vi "Main.vi"() -> ()   [LabVIEW 2017]
doc: "The myRIO Project template acquires acceleration data from the onboard accelerometer and displays the changes of acceleration values in a waveform chart."
uses:
  <vilib>/myRIO/Instrument Drivers/Onboard IO/I2C/typedefs/I2C User Configuration.ctl
  <vilib>/myRIO/Instrument Drivers/Onboard IO/I2C/typedefs/I2C Transfer Rate.ctl
  <vilib>/Platform/TimedLoop/XDataNode/timing_clust.ctl
  <vilib>/Platform/TimedLoop/XDataNode/nitl_modes.ctl
  <vilib>/Platform/TimedLoop/XDataNode/wakeup.ctl
  <vilib>/myRIO/Instrument Drivers/Onboard IO/DIO/typedefs/DIO Reference.ctl
  <vilib>/myRIO/Common/Instrument Driver Framework/Utilities/typedefs/myRIO Generic Hardware Reference.ctl
  <vilib>/myRIO/Common/Instrument Driver Framework/Utilities/typedefs/Hardware Version Enum.ctl
  <vilib>/myRIO/Common/Instrument Driver Framework/Utilities/typedefs/myRIO v1.0 Reference.ctl
  <vilib>/myRIO/Common/Instrument Driver Framework/Utilities/typedefs/Generic FPGA Reference.ctl
  <vilib>/myRIO/Common/Instrument Driver Framework/myRIO v1.0/DIO/typedefs/DIO Channels List.ctl
  <vilib>/myRIO/Common/Instrument Driver Framework/myRIO v1.0/DIO/typedefs/DIO Channels Enum.ctl
  <vilib>/userdefined/High Color/nirio_resource_hc.ctl
  <vilib>/myRIO/Common/Instrument Driver Framework/myRIO v1.0/Encoder/typedefs/Encoder Signal Mode.ctl
  <vilib>/myRIO/Instrument Drivers/Onboard IO/Encoder/typedefs/Encoder Reference.ctl
  <vilib>/myRIO/Common/Instrument Driver Framework/myRIO v1.0/Encoder/typedefs/Encoder Channels Enum.ctl
  <vilib>/myRIO/Common/Instrument Driver Framework/myRIO v1.0/Encoder/typedefs/Encoder Configuration v1.0.ctl
  <vilib>/myRIO/Instrument Drivers/Onboard IO/PWM/typedefs/PWM Reference.ctl
  <vilib>/myRIO/Common/Instrument Driver Framework/myRIO v1.0/PWM/typedefs/PWM Channels Enum.ctl
  <vilib>/myRIO/Instrument Drivers/Onboard IO/PWM/typedefs/PWM Configuration.ctl
  <vilib>/myRIO/Common/Instrument Driver Framework/Utilities/vis/Is FPGA Ref Available.vi
  <vilib>/myRIO/Common/Instrument Driver Framework/myRIO v1.0/Encoder/vis/myRIO v1.1 Open Encoder.vi
  <vilib>/myRIO/Common/Instrument Driver Framework/myRIO v1.0/DIO/vis/myRIO v1.1 Open DIO.vi
  <vilib>/myRIO/Common/Instrument Driver Framework/myRIO v1.0/PWM/vis/myRIO v1.1 Open PWM.vi
  <vilib>/myRIO/Instrument Drivers/Onboard IO/PWM/vis/Set Duty Cycle and Frequency.vi
  <vilib>/myRIO/Common/Instrument Driver Framework/Utilities/vis/Validate Channels.vi
  <vilib>/myRIO/Common/Instrument Driver Framework/myRIO v1.0/Encoder/vis/myRIO v1.0 Reserve Encoder.vi
  <vilib>/myRIO/Common/Instrument Driver Framework/myRIO v1.0/DIO/vis/myRIO v1.0 Reserve DIO.vi
  <vilib>/myRIO/Common/Instrument Driver Framework/myRIO v1.0/PWM/vis/myRIO v1.0 Reserve PWM.vi
  <vilib>/myRIO/Common/Instrument Driver Framework/myRIO v1.0/UART/vis/myRIO v1.0 Close UART.vi
  <vilib>/myRIO/Common/Instrument Driver Framework/myRIO v1.0/I2C/vis/myRIO v1.1 Open I2C.vi
  <vilib>/myRIO/Common/Instrument Driver Framework/myRIO v1.0/Encoder/vis/myRIO v1.0 Build MUX Configuration Encoder.vi
  <vilib>/myRIO/Common/Instrument Driver Framework/myRIO v1.0/Resource Manager/vis/myRIO v1.0 Reserve Channel List.vi
  <vilib>/myRIO/Common/Instrument Driver Framework/myRIO v1.0/DIO/vis/myRIO v1.0 Build MUX Configuration DIO.vi
  <vilib>/myRIO/Common/Instrument Driver Framework/myRIO v1.0/PWM/vis/myRIO v1.0 Build MUX Configuration PWM.vi
  <vilib>/myRIO/Common/Instrument Driver Framework/myRIO v1.0/I2C/vis/myRIO v1.0 Reserve I2C.vi
  <vilib>/myRIO/Common/Instrument Driver Framework/myRIO v1.0/Resource Manager/vis/myRIO v1.0 Create Configuration List.vi
  <vilib>/myRIO/Common/Instrument Driver Framework/myRIO v1.0/Resource Manager/vis/myRIO v1.0 Reserve Channel.vi
  <vilib>/myRIO/Common/Instrument Driver Framework/myRIO v1.0/Resource Manager/vis/myRIO v1.0 Unreserve Channel.vi
  <vilib>/myRIO/Common/Instrument Driver Framework/myRIO v1.0/I2C/vis/myRIO v1.0 Build MUX Configuration I2C.vi
  <vilib>/myRIO/Common/Instrument Driver Framework/myRIO v1.0/Resource Manager/vis/myRIO v1.0 Build Mutex Name.vi
  <vilib>/Utility/VariantDataType/GetNumericInfo.vi
  <vilib>/Utility/error.llb/Error Cluster From Error Code.vi
  <vilib>/myRIO/Common/Instrument Driver Framework/myRIO v1.0/myRIO v1.1 Open.vi
  <vilib>/myRIO/Common/Instrument Driver Framework/Utilities/vis/IO Manager.vi
  <vilib>/myRIO/Common/Instrument Driver Framework/Utilities/vis/Configuration Manager.vi
  <vilib>/myRIO/Common/Instrument Driver Framework/myRIO v1.0/Resource Manager/vis/myRIO v1.0 Configure IO.vi
  <vilib>/myRIO/Common/Instrument Driver Framework/myRIO v1.0/myRIO v1.0 Close.vi
  <vilib>/myRIO/Common/Instrument Driver Framework/myRIO v1.0/I2C/vis/myRIO v1.0 Configure I2C.vi
  <vilib>/myRIO/Common/Instrument Driver Framework/myRIO v1.0/I2C/vis/myRIO v1.0 Write I2C.vi
  <vilib>/myRIO/Common/Instrument Driver Framework/myRIO v1.0/DIO/vis/myRIO v1.0 Read DIO.vi
  <vilib>/myRIO/Common/Instrument Driver Framework/myRIO v1.0/DIO/vis/myRIO v1.0 Write DIO.vi
  <vilib>/myRIO/Common/Instrument Driver Framework/myRIO v1.0/I2C/vis/myRIO v1.0 Read I2C.vi
  <vilib>/myRIO/Common/Instrument Driver Framework/Utilities/vis/FPGA Ref Manager.vi
  <vilib>/myRIO/Common/Instrument Driver Framework/myRIO v1.0/myRIO v1.0 Reset FPGA.vi
  <vilib>/myRIO/Common/Instrument Driver Framework/myRIO v1.0/IRQ/vis/myRIO v1.0 IRQ Info FGV.vi
  <vilib>/myRIO/Common/Instrument Driver Framework/myRIO v1.0/IRQ/vis/myRIO v1.0 Timer IRQ Info FGV.vi
  <vilib>/myRIO/Common/Instrument Driver Framework/myRIO v1.0/IRQ/vis/myRIO v1.0 ISR Agent.vi
  <vilib>/myRIO/Common/Instrument Driver Framework/myRIO v1.0/Encoder/vis/myRIO v1.0 Configure Encoder.vi
  <vilib>/myRIO/Common/Instrument Driver Framework/myRIO v1.0/Encoder/vis/myRIO v1.0 Read Encoder.vi
  <vilib>/myRIO/Common/Instrument Driver Framework/myRIO v1.0/PWM/vis/myRIO v1.0 Write PWM.vi
  <vilib>/platform/TimedLoop/XDataNode/XDataNode.xnode
  <vilib>/myRIO/Express VI/Onboard IO/DO/DO Express VI.xnode
  <vilib>/myRIO/Instrument Drivers/Onboard IO/DIO/vis/myRIO DIO Open.xnode
  <vilib>/myRIO/Express VI/Onboard IO/Encoder/Encoder Express VI.xnode
  <vilib>/myRIO/Common/Instrument Driver Framework/myRIO v1.0/Encoder/typedefs/Encoder Count Direction Enum.ctl
  <vilib>/myRIO/Instrument Drivers/Onboard IO/Encoder/vis/myRIO Encoder Open.xnode
  <vilib>/myRIO/Express VI/Onboard IO/PWM/PWM Express VI.xnode
  <vilib>/myRIO/Instrument Drivers/Onboard IO/PWM/vis/myRIO PWM Open.xnode
  <vilib>/myRIO/Instrument Drivers/Utilities/Utilities.lvlib
  <vilib>/myRIO/Instrument Drivers/Onboard IO/I2C/I2C.lvlib
  <vilib>/myRIO/Instrument Drivers/Onboard IO/DIO/DIO.lvlib
  <vilib>/Platform/TimedLoop/XDataNode/XDNodeRunTimeDep.lvlib
  <vilib>/ptbypt/NI_PtbyPt.lvlib
  <vilib>/myRIO/Instrument Drivers/Onboard IO/Encoder/Encoder.lvlib
  <vilib>/myRIO/Instrument Drivers/Onboard IO/PWM/PWM.lvlib
panel:
  out "Led":bool
  in  "[ESC]":bool
  out "X":i16
  out "Y":i16
  out "Z":i16
  out "DATA":u8[](array[numeric]) format="%02x"
  out "Waveform Chart":cluster{i16, i16, i16}(graph)
  out "INT_SOURCE":bool[](array[boolean])
  out "error out":errorcluster
  in  "Stop":bool
  in  "(PWM Duty %)":dbl(slide)=1.0 scale=1.0..0.3
  in  "Direction":bool caption="Dirección"
  in  "Reseteo del contador":bool
  out "Contador":i32 format="%1d"
  out "Dirección":enum16{"Counting Up", "Counting Down"}(ring)
  in  "[ESC] 2":bool
  out "X rate":i16
  out "Y rate":i16
  out "Z rate":i16
  out "DATA 2":u8[](array[numeric]) format="%02x"
  out "Angular rate [LSB/sec]":cluster{i16, i16, i16}(graph)
  out "Angular displacement [LSB]":T1(graph)
  out "X displacement":dbl format="%#_5g"
  out "Y displacement":dbl format="%#_5g"
  out "Z displacement":dbl format="%#_5g"
  in  "reset integrator":bool
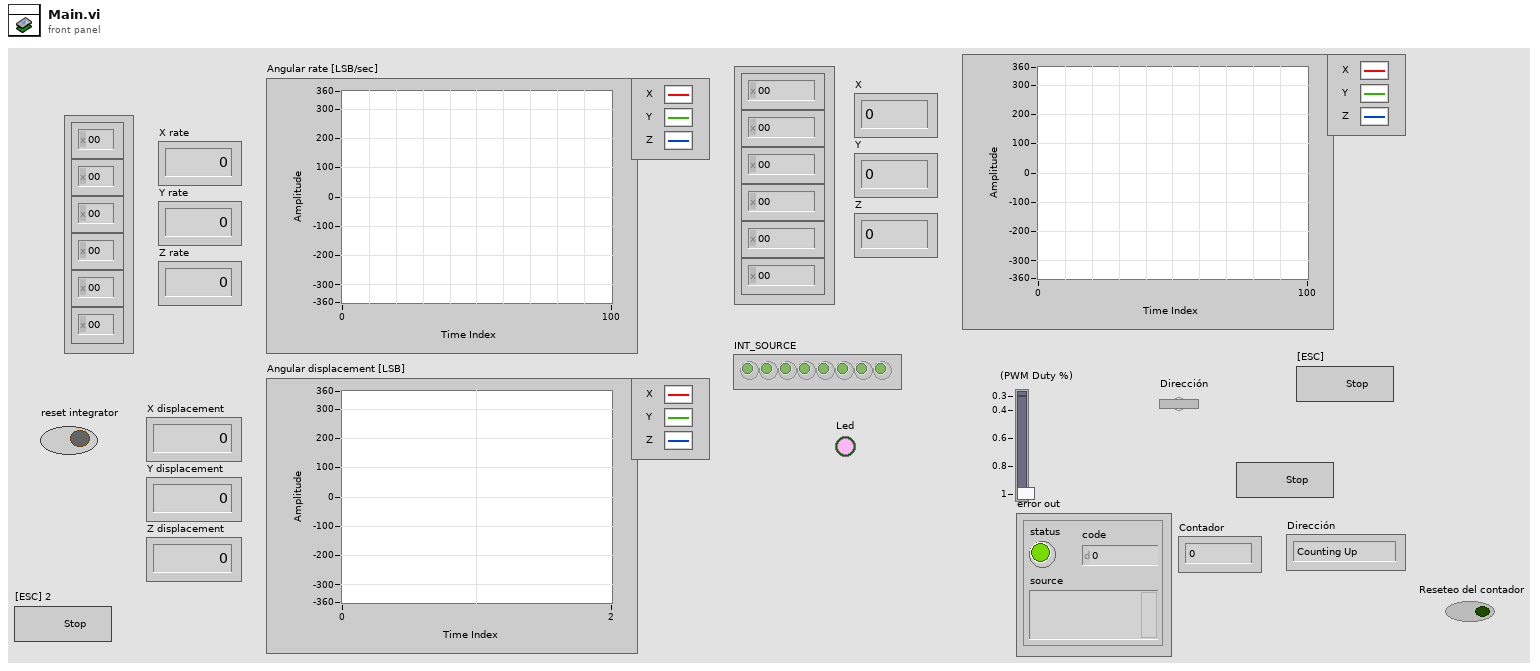
[diagram p1: front panel]
types:
  T1 = cluster{"integral x(t)":dbl, "integral x(t)":dbl, "integral x(t)":dbl}
  T2 = typedef "I2C.lvlib/I2C User Configuration.ctl" = cluster{"I2C Transfer Rate":T3}
  T3 = typedef "I2C.lvlib/I2C Transfer Rate.ctl" = enum16{"Standard mode (100 kbps)", "Fast mode (400 kbps)"}
  T4 = typedef "Encoder.lvlib/Encoder Reference.ctl" = cluster{"myRIO Reference":T5, "Encoder Channels Enum":T9}
  T5 = typedef "myRIO Generic Hardware Reference.ctl" = cluster{"myRIO Model":T6, "myRIO Hardware Reference":T7}
  T6 = typedef "Hardware Version Enum.ctl" = enum16{"Unknown", "myRIO-1900", "myRIO-1950", "roboRIO", "NI ELVIS RIO CM"}
  T7 = typedef "myRIO v1.0 Reference.ctl" = cluster{"Generic FPGA Reference":T8, "Allow multiple opens":bool}
  T8 = typedef "Generic FPGA Reference.ctl" = refnum<k20>
  T9 = typedef "Encoder Channels Enum.ctl" = enum16{"Not Connected", "C/ENC0", "C/ENC1", "A/ENC", "B/ENC", "DIO/ENC0", "DIO/ENC1", "DIO/ENC2", "DIO/ENC3", "DIO/ENC4"}
  T10 = typedef "Encoder Signal Mode.ctl" = enum16{"Quadrature phase signal", "Step and direction signal"}
  T11 = typedef "nirio_resource_hc.ctl" = tag
  T12 = typedef "DIO.lvlib/DIO Reference.ctl" = cluster{"myRIO Reference":T5, "DIO Channels List":T13}
  T13 = typedef "DIO Channels List.ctl" = T14[]
  T14 = typedef "DIO Channels Enum.ctl" = enum16{"Not Connected", "C/DIO0", "C/DIO1", "C/DIO2", "C/DIO3", "C/DIO4", "C/DIO5", "C/DIO6", "C/DIO7", "A/DIO0", "A/DIO1", "A/DIO2", "A/DIO3", "A/DIO4", "A/DIO5", "A/DIO6", "A/DIO7", "A/DIO8", "A/DIO9", "A/DIO10", "A/DIO11", "A/DIO12", "A/DIO13", "A/DIO14", "A/DIO15", "B/DIO0", "B/DIO1", "B/DIO2", "B/DIO3", "B/DIO4", "B/DIO5", "B/DIO6", "B/DIO7", "B/DIO8", "B/DIO9", "B/DIO10", "B/DIO11", "B/DIO12", "B/DIO13", "B/DIO14", "B/DIO15", "LED0", "LED1", "LED2", "LED3", "Button0", "DIO/DIO0", "DIO/DIO1", "DIO/DIO2", "DIO/DIO3", "DIO/DIO4", "DIO/DIO5", "DIO/DIO6", "DIO/DIO7", "DIO/DIO8", "DIO/DIO9", "SPI/CS0", "SPI/CS1", "SPI/CS2", "SPI/CS3", "LED RADIO (Green)", "LED RADIO (Red)", "LED COMM (Green)", "LED COMM (Red)", "LED MODE (Green)", "LED MODE (Red)"}
  T15 = typedef "PWM.lvlib/PWM Reference.ctl" = cluster{"myRIO Reference":T5, "PWM Channels Enum":T16, "PWM Configuration":T17}
  T16 = typedef "PWM Channels Enum.ctl" = enum16{"Not Connected", "C/PWM0", "C/PWM1", "A/PWM0", "A/PWM1", "A/PWM2", "B/PWM0", "B/PWM1", "B/PWM2", "PWM/PWM0", "PWM/PWM1", "PWM/PWM2", "PWM/PWM3", "PWM/PWM4", "PWM/PWM5", "PWM/PWM6", "PWM/PWM7", "PWM/PWM8", "PWM/PWM9"}
  T17 = typedef "PWM.lvlib/PWM Configuration.ctl" = cluster{"Frequency":dbl, "Duty Cycle":dbl}
  T18 = typedef "Encoder Count Direction Enum.ctl" = enum16{"Counting Up", "Counting Down"}
  T19 = typedef "I2C.lvlib/I2C Reference.ctl" = cluster{"myRIO Reference":T5, "I2C Channels Enum":T20, "I2C Configuration":T21}
  T20 = typedef "I2C Channels Enum.ctl" = enum16{"Not Connected", "A/I2C", "B/I2C", "I2C/I2C"}
  T21 = typedef "I2C.lvlib/I2C Configuration.ctl" = cluster{"I2C Transfer Rate":T3}
  T22 = typedef "XDNodeRunTimeDep.lvlib/timing_clust.ctl" = cluster{"Expected End [f-1]":u64, "Actual End [f-1]":u64, "Finished Late? [f-1]":bool, "Expected End [i-1]":u64, "Actual End [i-1]":u64, "Finished Late? [i-1]":bool, "Expected Start [i]":u64, "Actual Start [i]":u64, "Expected Start [f]":u64, "Actual Start [f]":u64, "Source Name":string, "Structure Name":string, "Period":i64, "Deadline":i64, "Offset":i64, "Start":i64, "Priority":i32, "Timeout":i32, "Mode":T23, "Wakeup Reason":T24, "Error":errorcluster, "Source Type":string, "Secondary Source Type":string, "Global End Time":u64, "Global Start Time":u64, "Frame Duration":u64, "Iteration Duration":u64, "Assigned CPU":i32, "I/O Scan Engine Mode":u32}
  T23 = typedef "XDNodeRunTimeDep.lvlib/nitl_modes.ctl" = enum32{"No Change", "Process missed periods, maintain original phase", "Discard missed periods, maintain original phase", "Process missed periods, ignore original phase", "Discard missed periods, ignore original phase"}
  T24 = typedef "XDNodeRunTimeDep.lvlib/wakeup.ctl" = enum32{"Normal", "Aborted", "Asynchronous wakeup", "Timing source error", "Timed loop error", "Timeout"}
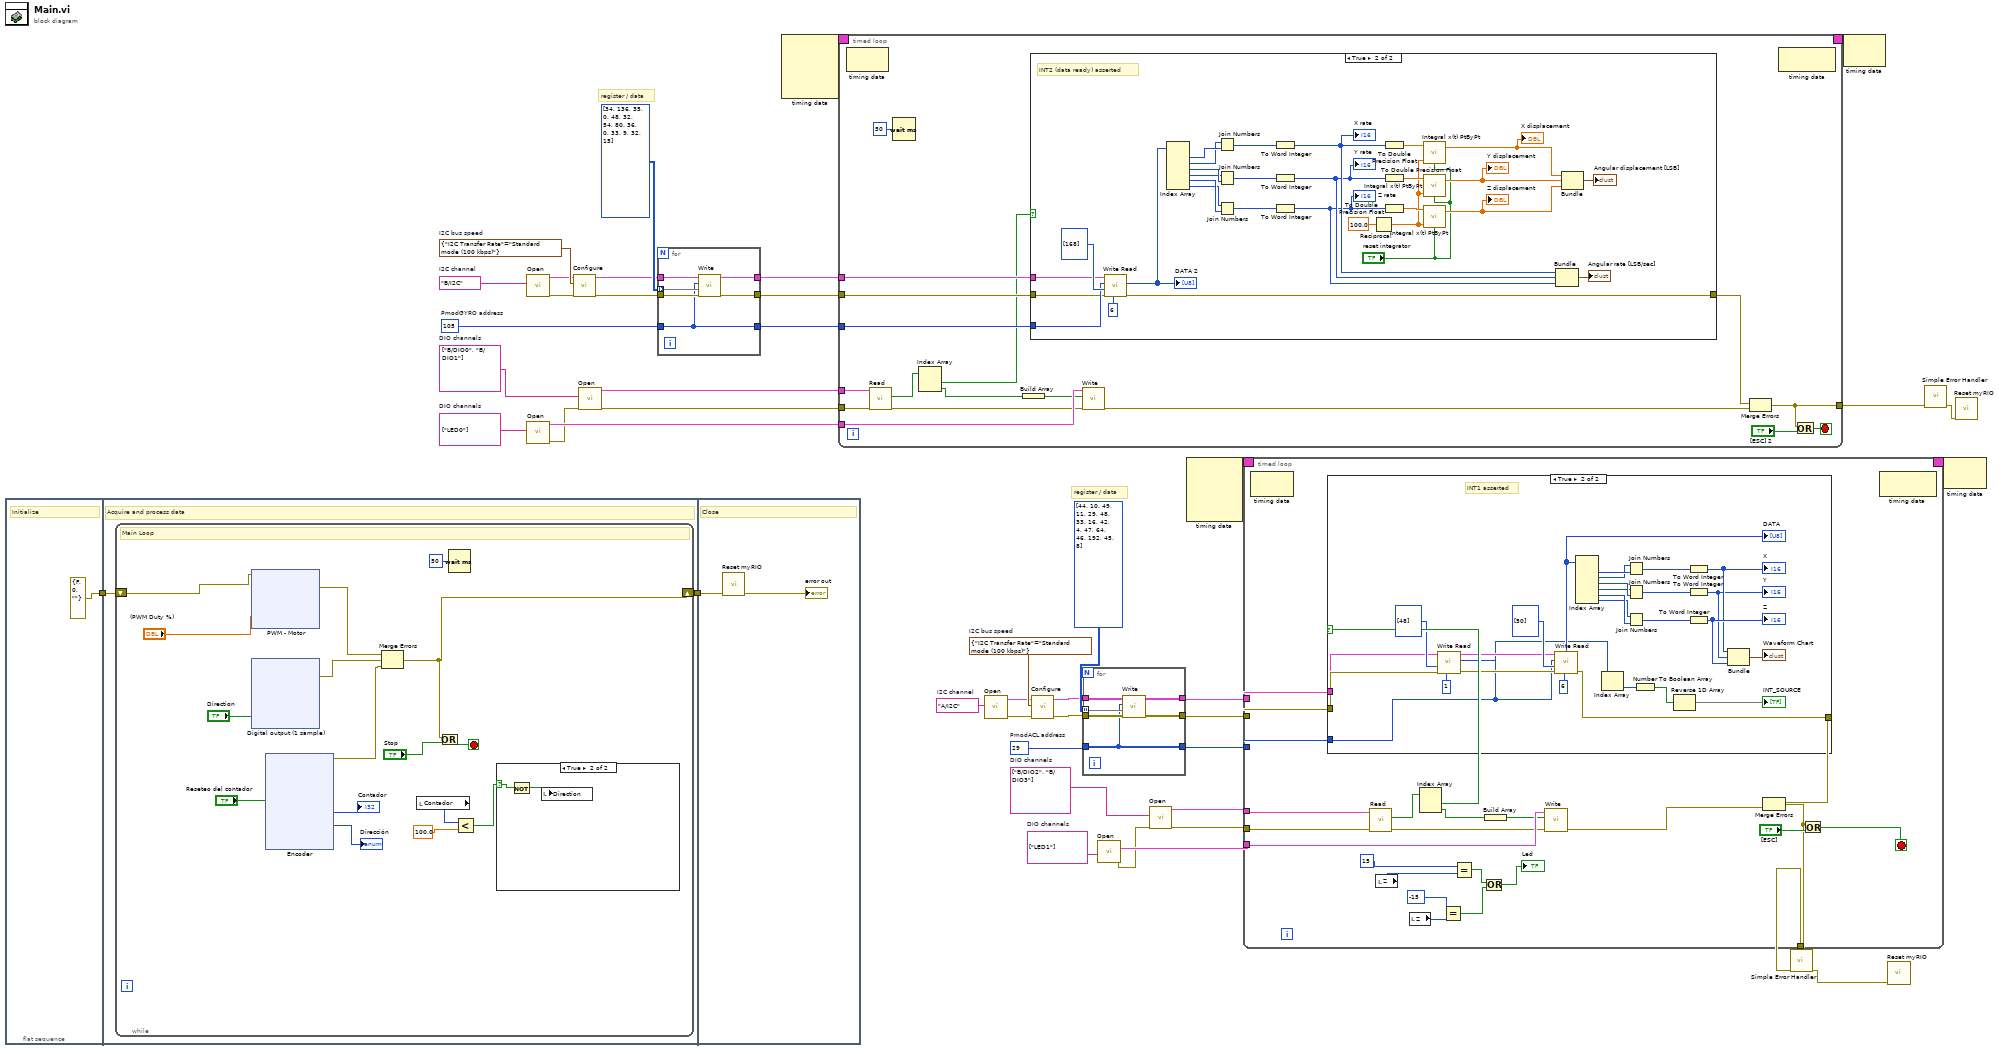
[diagram p0: block diagram]
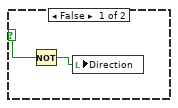
[diagram p3: hidden frame]
diagram:
  w3 = tag[] ["LED1"]  # DIO channels
  w4 = tag[] ["B/DIO2", "B/DIO3"]  # DIO channels
  w16 = T2 {"I2C Transfer Rate"=enum."Standard mode (100 kbps)"}  # I2C bus speed
  w17 = tag "A/I2C"  # I2C channel
  w7 = u8 29  # PmodACL address
  w26 = tag[] ["LED0"]  # DIO channels
  w27 = tag[] ["B/DIO0", "B/DIO1"]  # DIO channels
  w39 = T2 {"I2C Transfer Rate"=enum."Standard mode (100 kbps)"}  # I2C bus speed
  w40 = tag "B/I2C"  # I2C channel
  w30 = u8 105  # PmodGYRO address
  # "register / data"
  # "register / data"
  n1 = flat-sequence {
    tunnel: [errorcluster {"status"=FALSE, "code"=0, "source"=""} ("error in (no error)")] -> w23
    tunnel: w23 -> [w47]
    tunnel: [w46] -> w22
    tunnel: w22 -> [w185]
    frame #0 {
      # "Initialize"
    }
    frame #1 {
      # "Acquire and process data"
      n2 = while {
        shift-right: [w57] -> w46
        shift-left: w47 -> [w60]
        stop <- w62 stop-if-true
        # "Main Loop"
        n3 = xnode "PWM - Motor"("Duty Cycle"="(PWM Duty %)", "error in (no error)"=w60) -> ("error out"=w59:errorcluster)
        n4 = xnode "Digital output (1 sample)"("DIR0 (A/DIO6 (Pin 23))"="Direction") -> ("error out"=w58:errorcluster)  [unwired: 1 in]
        n5 = xnode "Encoder"("Reset Counter"="Reseteo del contador") -> ("Counter Value"=→"Contador":i32, "Counter Direction"=→"Dirección":T18, "error out"=w55:errorcluster)  [unwired: 1 in, 1 out]
        n6 = Merge Errors(w59, w58, w55) -> (w57:errorcluster)
        n7 = local read "Contador"() -> (w50:i32)
        n8 = Or(x=w57, y="Stop") -> (x .or. y?=w62:bool)
        n9 = Wait (ms)(milliseconds to wait=u32 50) -> ()  [unwired: 1 out]
        n10 = Less?(x=w50, y=100.0) -> (x < y?=w49:bool)
        n11 = case shown="True" w49 {
          selector: w49 -> [w64 w67]
          frame False {
            n12 = Not(x=w64) -> (.not. x?=w65:bool)
            n13 = local write "Direction"(w65) -> ()
          }
          frame True {
            n14 = Not(x=w67) -> (.not. x?=w66:bool)
            n15 = local write "Direction"(w66) -> ()
          }
        }
      }
    }
    frame #2 {
      # "Close"
      n16 = call <vilib>:"Reset myRIO.vi"("error in (no error)"=w185) -> ("error out"=→"error out":errorcluster)  [unwired: 10 in]
    }
  }
  n17 = call <vilib>:"Open.vi"("Channel Name"=w40) -> ("error out"=w37:errorcluster, "I2C Ref Out"=w38:T19)  [unwired: 9 in]
  n18 = call <vilib>:"Open.vi"("Channel Names"=w26) -> ("error out"=w24:errorcluster, "DIO Ref Out"=w25:T12)  [unwired: 9 in]
  n19 = call <vilib>:"Configure.vi"("error in (no error)"=w37, "I2C User Configuration"=w39, "I2C Ref In"=w38) -> ("error out"=w31:errorcluster, "I2C Ref Out"=w32:T19)  [unwired: 7 in]
  n20 = call <vilib>:"Open.vi"("error in (no error)"=w24, "Channel Names"=w27) -> ("error out"=w29:errorcluster, "DIO Ref Out"=w28:T12)  [unwired: 8 in]
  n21 = for {
    tunnel: [w191] -> w36
    tunnel: [w190] -> w35
    tunnel: [w186] -> w34
    tunnel: u8[][] [[34, 136], [35, 0], [48, 32], [54, 80], [36, 0], [33, 9], [32, 15]] ("Bytes to Write") -> [w189] mode=indexing
    tunnel: w32 -> [w188]
    tunnel: w31 -> [w187]
    tunnel: w30 -> [w186]
    n22 = call <vilib>:"Write.vi"("error in (no error)"=w187, "Bytes to Write"=w189, "Slave Address (7-bit)"=w186, "I2C Ref In"=w188) -> ("error out"=w191:errorcluster, "I2C Ref Out"=w190:T19)  [unwired: 6 in]
  }
  n23 = node-c288() -> (w44:T22)  [unwired: 4 in]
  n24 = timed-loop {
    tunnel: [w193] -> w41
    tunnel: w34 -> [w204]
    tunnel: w36 -> [w206]
    tunnel: w35 -> [w205]
    tunnel: w29 -> [w203]
    tunnel: w28 -> [w202]
    timing: w44 -> [_]
    timing-out: [_] -> w43
    tunnel: w25 -> [w198]
    stop <- w208 stop-if-true
    n25 = node-c288() -> ()  [unwired: 1 in, 1 out]
    n26 = call <vilib>:"Read.vi"("error in (no error)"=w203, "DIO Ref In"=w202) -> ("error out"=w197:errorcluster, "Values"=w199:bool[])  [unwired: 7 in, 1 out]
    n27 = Wait (ms)(milliseconds to wait=u32 50) -> ()  [unwired: 1 out]
    n28 = Index Array "Index Array"(array=w199) -> (element #1=w200:bool, element #2=w195:bool)  [unwired: 2 in]
    n29 = Build Array "Build Array"(w195) -> (w196:bool[])
    n30 = case shown="True" w200 {
      tunnel: w206 -> [w211 w219]
      tunnel: w205 -> [_ w220]
      tunnel: w204 -> [_ w229]
      tunnel: [w211 w228] -> w201
      frame False {
        # "INT2 (data ready) deasserted"
      }
      frame True {
        # "INT2 (data ready) asserted"
        n31 = call <vilib>:"Write Read.vi"("Byte Count"=u32 6, "error in (no error)"=w219, "Bytes to Write"=u8[] [168], "Slave Address (7-bit)"=w229, "I2C Ref In"=w220) -> ("error out"=w228:errorcluster, "Bytes Read"=w227:u8[])  [unwired: 3 in, 1 out]
        "DATA 2" <- w227
        n32 = Index Array "Index Array"(array=w227) -> (element #1=w237:u8, element #2=w236:u8, element #3=w235:u8, element #4=w234:u8, element #5=w233:u8, element #6=w232:u8)  [unwired: 6 in]
        n33 = Join Numbers(hi=w236, lo=w237) -> ((hi.lo)=w241:u16)
        n34 = Join Numbers(hi=w234, lo=w235) -> ((hi.lo)=w240:u16)
        n35 = Join Numbers(hi=w232, lo=w233) -> ((hi.lo)=w239:u16)
        n36 = To Word Integer(number=w241) -> (16bit integer=w226:i16)
        "X rate" <- w226
        n37 = To Word Integer(number=w240) -> (16bit integer=w222:i16)
        "Y rate" <- w222
        n38 = To Word Integer(number=w239) -> (16bit integer=w221:i16)
        "Z rate" <- w221
        n39 = Reciprocal(x=100.0 ("dt")) -> (1/x=w217:dbl)
        n40 = To Double Precision Float(number=w226) -> (double precision float=w212:dbl)
        n41 = To Double Precision Float(number=w222) -> (double precision float=w225:dbl)
        n42 = To Double Precision Float(number=w221) -> (double precision float=w224:dbl)
        n43 = call <vilib>:"Integral x(t) PtByPt.vi"("initialize"="reset integrator", "dt"=w217, "x"=w212) -> ("integral x(t)"=w213:dbl)  [unwired: 1 in, 1 out]
        "X displacement" <- w213
        n44 = call <vilib>:"Integral x(t) PtByPt.vi"("initialize"="reset integrator", "dt"=w217, "x"=w225) -> ("integral x(t)"=w216:dbl)  [unwired: 1 in, 1 out]
        "Y displacement" <- w216
        n45 = call <vilib>:"Integral x(t) PtByPt.vi"("initialize"="reset integrator", "dt"=w217, "x"=w224) -> ("integral x(t)"=w215:dbl)  [unwired: 1 in, 1 out]
        "Z displacement" <- w215
        n46 = Bundle "Bundle"(w226, w222, w221) -> (→"Angular rate [LSB/sec]":cluster{i16, i16, i16})  [unwired: 1 in]
        n47 = Bundle "Bundle"("integral x(t)"=w213, "integral x(t)"=w216, "integral x(t)"=w215) -> (→"Angular displacement [LSB]":T1)  [unwired: 1 in]
      }
    }
    n48 = call <vilib>:"Write.vi"("error in (no error)"=w197, "Values"=w196, "DIO Ref In"=w198) -> ("error out"=w194:errorcluster)  [unwired: 6 in, 1 out]
    n49 = Merge Errors "Merge Errors"(w201, w194) -> (w193:errorcluster)
    n50 = node-c288() -> ()  [unwired: 1 in, 1 out]
    n51 = Or(x=w193, y="[ESC] 2") -> (x .or. y?=w208:bool)
  }
  n52 = call <vilib>:"Open.vi"("Channel Name"=w17) -> ("error out"=w14:errorcluster, "I2C Ref Out"=w15:T19)  [unwired: 9 in]
  n53 = call <vilib>:"Configure.vi"("error in (no error)"=w14, "I2C User Configuration"=w16, "I2C Ref In"=w15) -> ("error out"=w8:errorcluster, "I2C Ref Out"=w9:T19)  [unwired: 7 in]
  n54 = for {
    tunnel: [w247] -> w13
    tunnel: [w246] -> w12
    tunnel: [w242] -> w11
    tunnel: u8[][] [[44, 10], [49, 11], [29, 48], [33, 16], [42, 4], [47, 64], [46, 192], [45, 8]] ("Bytes to Write") -> [w245] mode=indexing
    tunnel: w9 -> [w244]
    tunnel: w8 -> [w243]
    tunnel: w7 -> [w242]
    n55 = call <vilib>:"Write.vi"("error in (no error)"=w243, "Bytes to Write"=w245, "Slave Address (7-bit)"=w242, "I2C Ref In"=w244) -> ("error out"=w247:errorcluster, "I2C Ref Out"=w246:T19)  [unwired: 6 in]
  }
  n56 = call <vilib>:"Open.vi"("Channel Names"=w3) -> ("error out"=w1:errorcluster, "DIO Ref Out"=w2:T12)  [unwired: 9 in]
  n57 = call <vilib>:"Open.vi"("error in (no error)"=w1, "Channel Names"=w4) -> ("error out"=w6:errorcluster, "DIO Ref Out"=w5:T12)  [unwired: 8 in]
  n58 = node-c288() -> (w21:T22)  [unwired: 4 in]
  n59 = timed-loop {
    tunnel: [w255] -> w18
    tunnel: w11 -> [w266]
    tunnel: w13 -> [w268]
    tunnel: w12 -> [w267]
    tunnel: w6 -> [w265]
    tunnel: w5 -> [w264]
    timing: w21 -> [_]
    timing-out: [_] -> w20
    tunnel: w2 -> [w260]
    stop <- w270 stop-if-true
    n60 = node-c288() -> ()  [unwired: 1 in, 1 out]
    n61 = call <vilib>:"Read.vi"("error in (no error)"=w265, "DIO Ref In"=w264) -> ("error out"=w259:errorcluster, "Values"=w261:bool[])  [unwired: 7 in, 1 out]
    n62 = local read "Z"() -> (w254:i16)
    n63 = local read "Z"() -> (w252:i16)
    n64 = Index Array "Index Array"(array=w261) -> (element #1=w262:bool, element #2=w257:bool)  [unwired: 2 in]
    n65 = case shown="True" w262 {
      tunnel: w268 -> [w273 w292]
      tunnel: w267 -> [_ w291]
      tunnel: w266 -> [_ w280]
      tunnel: [w273 w276] -> w263
      frame False {
        # "INT1 deasserted"
      }
      frame True {
        # "INT1 asserted"
        n66 = call <vilib>:"Write Read.vi"("Byte Count"=u32 1, "error in (no error)"=w292, "Bytes to Write"=u8[] [48], "Slave Address (7-bit)"=w280, "I2C Ref In"=w291) -> ("error out"=w281:errorcluster, "Bytes Read"=w274:u8[], "I2C Ref Out"=w282:T19)  [unwired: 3 in]
        n67 = call <vilib>:"Write Read.vi"("Byte Count"=u32 6, "error in (no error)"=w281, "Bytes to Write"=u8[] [50], "Slave Address (7-bit)"=w280, "I2C Ref In"=w282) -> ("error out"=w276:errorcluster, "Bytes Read"=w275:u8[])  [unwired: 3 in, 1 out]
        "DATA" <- w275
        n68 = Index Array "Index Array"(array=w275) -> (element #1=w290:u8, element #2=w289:u8, element #3=w288:u8, element #4=w287:u8, element #5=w286:u8, element #6=w285:u8)  [unwired: 6 in]
        n69 = Index Array "Index Array"(array=w274) -> (element=w279:u8)  [unwired: 1 in]
        n70 = Join Numbers(hi=w289, lo=w290) -> ((hi.lo)=w301:u16)
        n71 = Join Numbers(hi=w287, lo=w288) -> ((hi.lo)=w300:u16)
        n72 = Join Numbers(hi=w285, lo=w286) -> ((hi.lo)=w299:u16)
        n73 = Number To Boolean Array(number=w279) -> (Boolean array=w278:bool[])
        n74 = Reverse 1D Array(array=w278) -> (reversed array=→"INT_SOURCE":bool[])
        n75 = To Word Integer(number=w301) -> (16bit integer=w296:i16)
        "X" <- w296
        n76 = To Word Integer(number=w300) -> (16bit integer=w295:i16)
        "Y" <- w295
        n77 = To Word Integer(number=w299) -> (16bit integer=w298:i16)
        "Z" <- w298
        n78 = Bundle "Bundle"(w296, w295, w298) -> (→"Waveform Chart":cluster{i16, i16, i16})  [unwired: 1 in]
      }
    }
    n79 = Equal?(x=i16 -15 ("y"), y=w252) -> (x = y?=w248:bool)
    n80 = Equal?(x=i16 15 ("y"), y=w254) -> (x = y?=w249:bool)
    n81 = Or(x=w249, y=w248) -> (x .or. y?=→"Led":bool)
    n82 = Build Array "Build Array"(w257) -> (w258:bool[])
    n83 = call <vilib>:"Write.vi"("error in (no error)"=w259, "Values"=w258, "DIO Ref In"=w260) -> ("error out"=w256:errorcluster)  [unwired: 6 in, 1 out]
    n84 = Merge Errors "Merge Errors"(w263, w256) -> (w255:errorcluster)
    n85 = Or(x=w255, y="[ESC]") -> (x .or. y?=w270:bool)
    n86 = node-c288() -> ()  [unwired: 1 in, 1 out]
  }
  n87 = call <vilib>:"Simple Error Handler.vi"("error in (no error)"=w18) -> ("error out"=w19:errorcluster)  [unwired: 4 in, 4 out]
  n88 = node-c288(w43) -> ()  [unwired: 1 out]
  n89 = call <vilib>:"Reset myRIO.vi"("error in (no error)"=w19) -> ()  [unwired: 10 in, 1 out]
  n90 = call <vilib>:"Simple Error Handler.vi"("error in (no error)"=w41) -> ("error out"=w42:errorcluster)  [unwired: 4 in, 4 out]
  n91 = node-c288(w20) -> ()  [unwired: 1 out]
  n92 = call <vilib>:"Reset myRIO.vi"("error in (no error)"=w42) -> ()  [unwired: 10 in, 1 out]
